vi "IntakeBegin.vi"(8 "error in (no error)":errorcluster) -> (0 "error out":errorcluster)   [LabVIEW 2023]
uses:
  <vilib>/Rock Robotics/WPI/ThirdParty/REV Robotics/REVLib/Typedef/Spark MAX Sensor Type.ctl
  <vilib>/Rock Robotics/WPI/ThirdParty/REV Robotics/REVLib/Typedef/Spark MAX Idle Mode.ctl
  <vilib>/Rock Robotics/WPI/ThirdParty/REV Robotics/REVLib/Typedef/Spark MAX Motor Type.ctl
  <vilib>/Rock Robotics/SystemInterfaces/DIO/FPGA_DIOChannel.ctl
  <vilib>/Rock Robotics/WPI/Switch/WPI_SwitchOpenLimit.vi
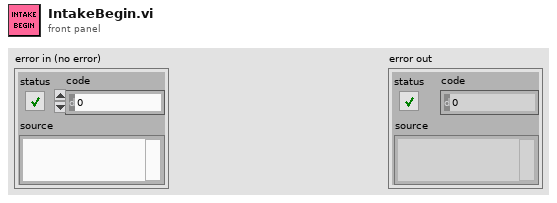
[diagram p1: front panel]
types:
  T1 = typedef "Spark MAX Sensor Type.ctl" = enum16{"No Sensor", "Hall Sensor", "Encoder", "-Not Available-", "Analog", "Alternate Encoder", "Duty Cycle"}
  T2 = typedef "Spark MAX Idle Mode.ctl" = enum16{"Coast", "Brake"}
  T3 = typedef "Spark MAX Motor Type.ctl" = enum16{"Brushed", "Brushless"}
  T4 = typedef "FPGA_DIOChannel.ctl" = enum8{"DIO 0", "DIO 1", "DIO 2", "DIO 3", "DIO 4", "DIO 5", "DIO 6", "DIO 7", "DIO 8", "DIO 9", "DIO MXP 0", "DIO MXP 1", "DIO MXP 2", "DIO MXP 3", "DIO MXP 4", "DIO MXP 5", "DIO MXP 6", "DIO MXP 7", "DIO MXP 8", "DIO MXP 9", "DIO MXP 10", "DIO MXP 11", "DIO MXP 12", "DIO MXP 13", "DIO MXP 14", "DIO MXP 15", "SPI Port CS1", "SPI Port CS2", "SPI Port CS3", "SPI Port MISO", "SPI Port MOSI", "Invalid"}
  T5 = typedef "WPI_MotorControlDeviceRef.ctl" = cluster{"DeviceStatus":errorcluster, "Type":T6, "PWM":cluster{"PWM Channel":T7, "DeadBand":T8}, "CAN":cluster{"Device Number":u8, "SetOutput VI Ref":variant, "GetOutput VI Ref":variant, "Enable VI Ref":variant, "Disable VI Ref":variant, "Data":variant}, "Invert":bool, "DIO PWM":cluster{"PWM \"Enable\" Channel":T7, "DIOChannel":T4, "PWM Rate":dbl}}
  T6 = typedef "WPI_MotorControlType.ctl" = enum16{"PWM", "CAN", "DIO PWM"}
  T7 = typedef "FPGA_DIOPWMChannel.ctl" = enum8{"PWM 0", "PWM 1", "PWM 2", "PWM 3", "PWM 4", "PWM 5", "PWM 6", "PWM 7", "PWM 8", "PWM 9", "PWM MXP 0", "PWM MXP 1", "PWM MXP 2", "PWM MXP 3", "PWM MXP 4", "PWM MXP 5", "PWM MXP 6", "PWM MXP 7", "PWM MXP 8", "PWM MXP 9", "Invalid"}
  T8 = typedef "WPI_PWMDeadband.ctl" = cluster{"Name":string, "maxPositivePwm":i32, "minPositivePwm":i32, "centerPwm":i32, "maxNegativePwm":i32, "minNegativePwm":i32, "angularRange":u16}
  T9 = typedef "WPI_SwitchDevRef.ctl" = cluster{"DevStatus":errorcluster, "DIO Channel":T4, "CntIndex":T10, "Normally Closed":bool}
  T10 = typedef "FPGA_CounterCtrSystemIndex.ctl" = enum8{"Ctr 0", "Ctr 1", "Ctr 2", "Ctr 3", "Ctr 4", "Ctr 5", "Ctr 6", "Ctr 7", "Invalid"}
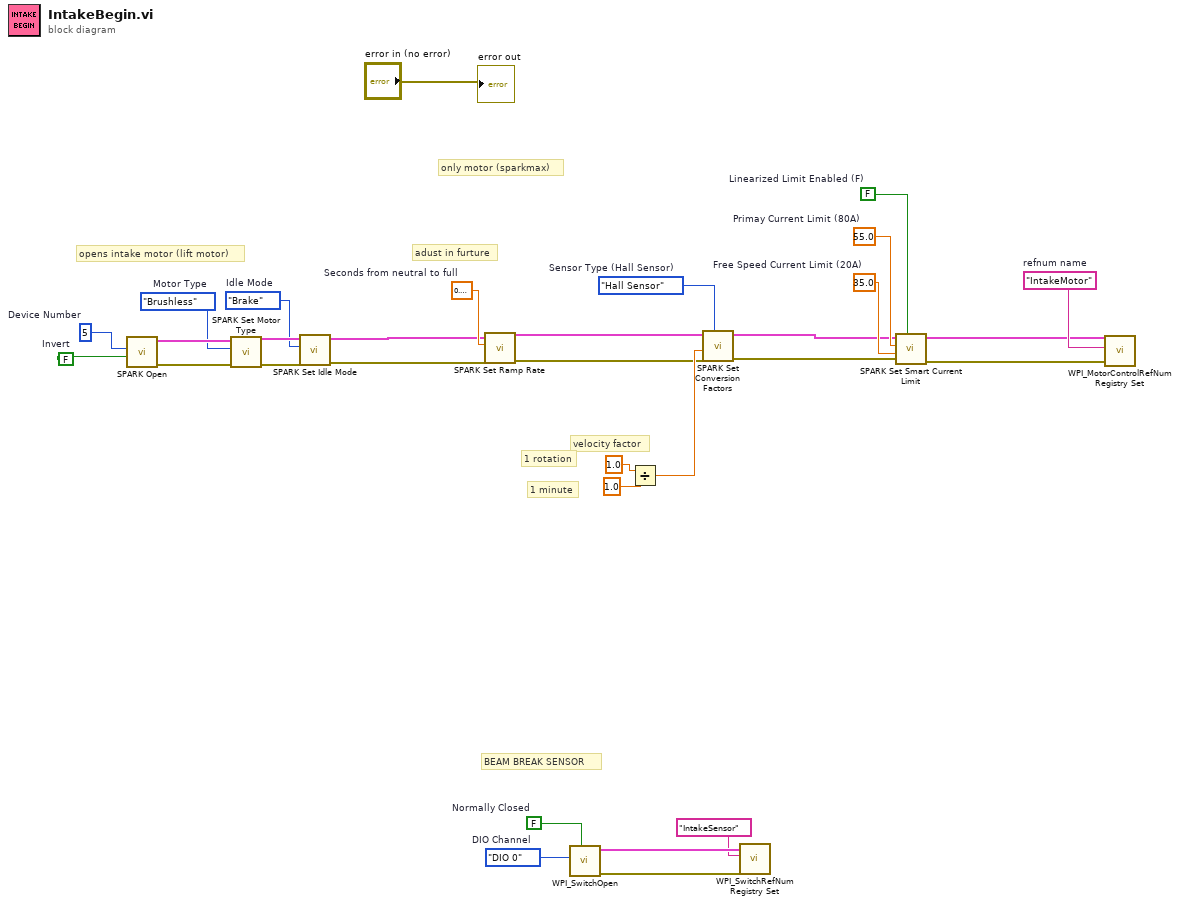
[diagram p0: block diagram]
diagram:
  w13 = FALSE  # Linearized Limit Enabled (F)
  w15 = Spark_MAX_Sensor_Type."Hall Sensor"  # Sensor Type (Hall Sensor)
  w17 = sgl 0.2  # Seconds from neutral to full
  w18 = "IntakeMotor"  # refnum name
  w19 = 35.0  # Free Speed Current Limit (20A)
  w20 = 55.0  # Primay Current Limit (80A)
  w21 = Spark_MAX_Idle_Mode."Brake"  # Idle Mode
  w23 = Spark_MAX_Motor_Type."Brushless"  # Motor Type
  w25 = FALSE  # Invert
  w26 = u8 5  # Device Number
  w30 = FPGA_DIOChannel."DIO 0"  # DIO Channel
  w31 = FALSE  # Normally Closed
  # "1 minute"
  # "1 rotation"
  # "adust in furture"
  # "velocity factor"
  # "opens intake motor (lift motor)"
  # "only motor (sparkmax)"
  # "BEAM BREAK SENSOR"
  n1 = call <vilib>:"SPARK Open.vi"("Invert"=w25, "Device Number"=w26) -> ("error out"=w6:errorcluster, "MotorControlDeviceRef"=w24:T5)  [unwired: 8 in]
  n2 = call <vilib>:"SPARK Set Motor Type.vi"("error in (no error)"=w6, "Motor Type"=w23, "MotorControlDevRef"=w24) -> ("error out"=w5:errorcluster, "MotorControlDeviceRef"=w22:T5)  [unwired: 7 in]
  n3 = call <vilib>:"SPARK Set Idle Mode.vi"("error in (no error)"=w5, "Idle Mode"=w21, "MotorControlDeviceRef in"=w22) -> ("error out"=w4:errorcluster, "MotorControlDeviceRef out"=w8:T5)  [unwired: 7 in]
  n4 = call <vilib>:"SPARK Set Ramp Rate.vi"("error in (no error)"=w4, "Seconds from neutral to full (0)"=w17, "MotorControlDeviceRef in"=w8) -> ("error out"=w3:errorcluster, "MotorControlDeviceRef"=w16:T5)  [unwired: 7 in]
  n5 = call-poly <vilib>:"WPI_SwitchOpen.vi"("Normally Closed"=w31, "DIO Channel"=w30) -> ("error out"=w28:errorcluster, "SwitchDevRef"=w29:T9)  [unwired: 8 in]
  n6 = Divide(x=1.0 ("Velocity Factor (1)"), y=1.0) -> (x/y=w9:dbl)
  n7 = call <vilib>:"SPARK Set Conversion Factors.vi"("Sensor Type (Hall Sensor)"=w15, "error in (no error)"=w3, "Velocity Factor (1)"=w9, "MotorControlDeviceRef in"=w16) -> ("error out"=w2:errorcluster, "MotorControlDeviceRef out"=w14:T5)  [unwired: 6 in]
  n8 = call <vilib>:"WPI_SwitchRefNum Registry Set.vi"("error in (no error)"=w28, "refnum name"="IntakeSensor", "SwitchDevRef"=w29) -> ()  [unwired: 7 in, 2 out]
  n9 = call <vilib>:"SPARK Set Smart Current Limit.vi"("Linearized Limit Enabled (F)"=w13, "error in (no error)"=w2, "Free Speed Current Limit (20A)"=w19, "Primay Current Limit (80A)"=w20, "MotorControlDeviceRef in"=w14) -> ("error out"=w1:errorcluster, "MotorControlDeviceRef out"=w7:T5)  [unwired: 5 in]
  n10 = call <vilib>:"WPI_MotorControlRefNum Registry Set.vi"("error in (no error)"=w1, "refnum name"=w18, "MotorControlDevRef"=w7) -> ()  [unwired: 7 in, 2 out]
  "error out" <- "error in (no error)"
